vi "USB.Get Enum Data based on Service.vi"(3 "Service":string) -> (1 "Enum Key Data":string[](array[string]))   [LabVIEW 2018]
uses:
  <vilib>/registry/registry.llb/Registry RtKey.ctl
  <vilib>/registry/registry.llb/Registry SAM.ctl
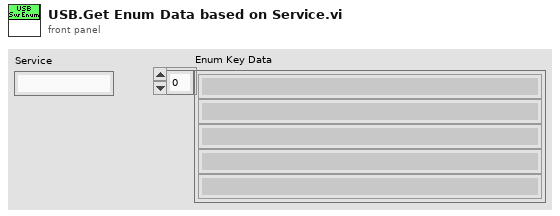
[diagram p1: front panel]
types:
  T1 = typedef "Registry SAM.ctl" = enum32{"KEY_QUERY_VALUE", "KEY_SET_VALUE", "KEY_CREATE_SUB_KEY", "KEY_ENUMERATE_SUB_KEYS", "KEY_NOTIFY", "KEY_CREATE_LINK", "KEY_READ", "KEY_WRITE", "KEY_ALL_ACCESS", "KEY_READ | KEY_WRITE"}
  T2 = typedef "Registry RtKey.ctl" = enum32{"HKEY_CLASSES_ROOT", "HKEY_CURRENT_USER", "HKEY_LOCAL_MACHINE", "HKEY_USERS", "HKEY_PERFORMANCE_DATA", "HKEY_CURRENT_CONFIG", "HKEY_DYN_DATA"}
  T3 = typedef "Registry refnum.ctl" = refnum<k1>
  T4 = cluster{"numValues":i32, "maxValueNameLen":i32, "maxValueDataLen":i32}
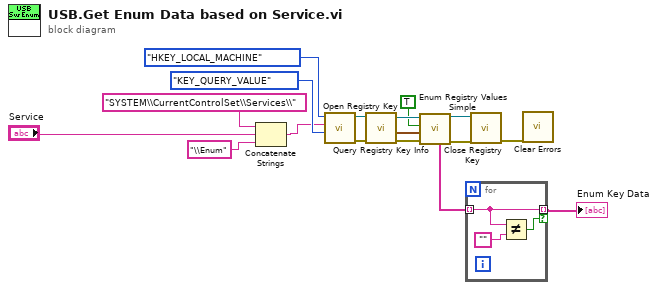
[diagram p0: block diagram]
diagram:
  n1 = Concatenate Strings("SYSTEM\\CurrentControlSet\\Services\\", "Service", "\\Enum") -> (w5:string)
  n2 = call <vilib>:"Open Registry Key.vi"("security access mask (KEY_READ | KEY_WRITE)"=Registry_SAM."KEY_QUERY_VALUE", "subkey"=w5, "root key (HKEY_LOCAL_MACHINE)"=Registry_RtKey."HKEY_LOCAL_MACHINE") -> ("error out"=w14:errorcluster, "refnum out"=w15:T3)  [unwired: 1 in, 6 out]
  n3 = call <vilib>:"Query Registry Key Info.vi"("error in (no error)"=w14, "refnum"=w15) -> ("error out"=w13:errorcluster, "value info"=w11:T4, "refnum out"=w12:T3)  [unwired: 7 out]
  n4 = call <vilib>:"Enum Registry Values Simple.vi"("error in (no error)"=w13, "value info"=w11, "retrieve data? (F)"=TRUE, "refnum"=w12) -> ("error out"=w8:errorcluster, "refnum out"=w9:T3, "String/Binary data"=w2:string[])  [unwired: 2 in, 3 out]
  n5 = for {
    tunnel: w2 -> [w19] mode=indexing
    tunnel: [w19] -> w1 mode=indexing if=w18
    n6 = Not Equal?(x=w19, y="") -> (x != y?=w18:bool)
  }
  "Enum Key Data" <- w1
  n7 = call <vilib>:"Close Registry Key.vi"("error in (no error)"=w8, "refnum"=w9) -> ("error out"=w4:errorcluster)  [unwired: 5 out]
  n8 = call <vilib>:"Clear Errors.vi"("error in (no error)"=w4) -> ()  [unwired: 5 in, 2 out]
